vi "Start_Stop.vi"(8 "error in (no error)":errorcluster, 10 "Start/Stop":bool, 11 "Aumentar_contador in":refnum<class "Aumentar_contador.lvclass">) -> (0 "error out":errorcluster, 3 "Aumentar_contador out":refnum<class "Aumentar_contador.lvclass">)   [LabVIEW 2019, in "Aumentar_contador.lvlib" / "Aumentar_contador.lvclass"]
uses:
  Aumentar_contador.lvclass
  Aumentar_contador.lvclass/Aumentar_contador.ctl
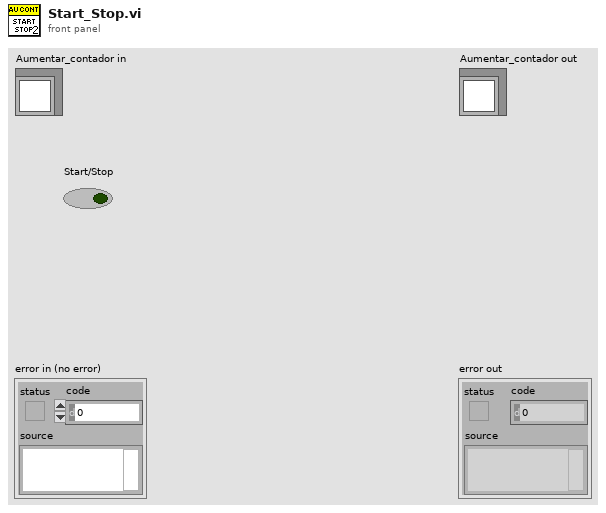
[diagram p1: front panel]
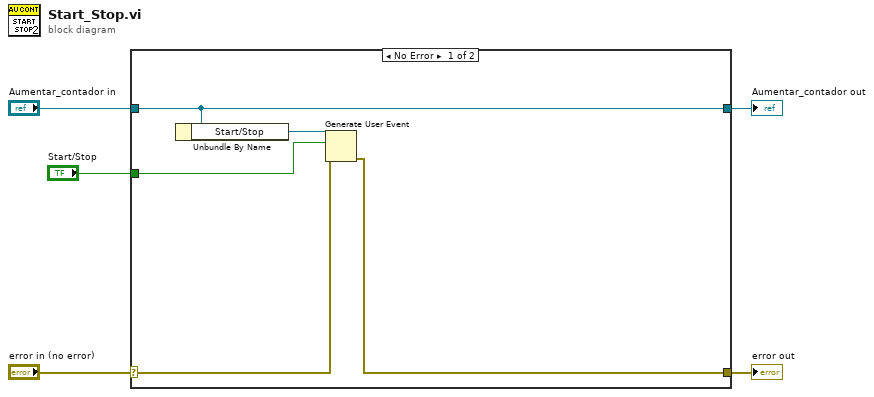
[diagram p0: block diagram]
diagram:
  n1 = case shown="No Error" "error in (no error)" {
    selector: "error in (no error)" -> [w7 w12]
    tunnel: [w6 w12] -> w4
    tunnel: [w10 w11] -> w2
    tunnel: "Aumentar_contador in" -> [w10 w11]
    tunnel: "Start/Stop" -> [w8 _]
    frame No Error {
      n2 = Unbundle By Name(w10) -> ("Start/Stop"=w9:refnum<user-event>)
      n3 = Generate User Event(user event=w9, event data cluster=w8, error in=w7) -> (error out=w6:errorcluster)  [unwired: 1 in, 1 out]
    }
    frame Error {
    }
  }
  "error out" <- w4
  "Aumentar_contador out" <- w2
